vi "MB Serial Call Wait on Query.vi"(9 "Timeout":u32=10000, 10 "Serial Parameters":T1 {"Slave Address" format="%.0x"}, 11 "VISA resource name":refnum<visa-resource-name>) -> ()   [LabVIEW 2011]
panel:
  # "VI Name: MB Serial Call Wait on Query.vi\nPurpose: Dynamically calls MB Serial Wait on Query.vi"
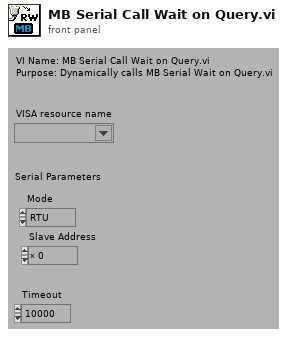
[diagram p1: front panel]
types:
  T1 = cluster{"Mode":enum16{"RTU", "ASCII"}, "Slave Address":u8}
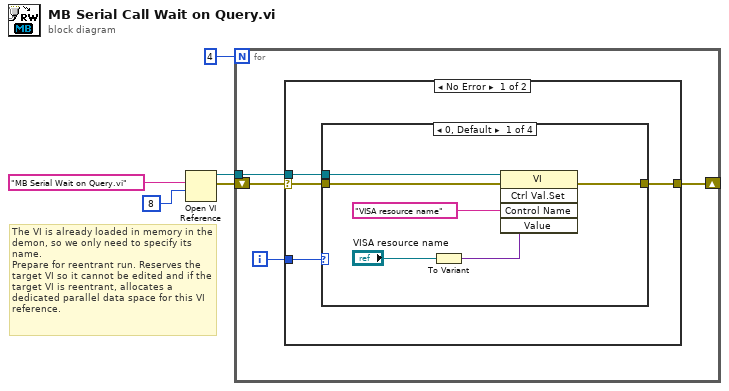
[diagram p0: block diagram]
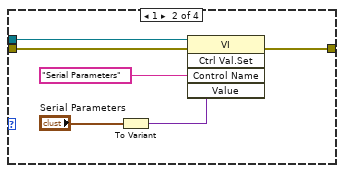
[diagram p2: hidden frame]
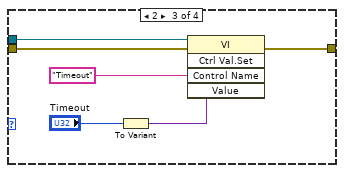
[diagram p3: hidden frame]
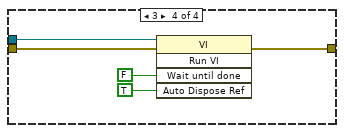
[diagram p4: hidden frame]
diagram:
  # "The VI is already loaded in memory in the demon, so we only need to specify its name.\nPrepare for reentrant run. Reserves the target VI so it cannot be edited and if the target VI is reentrant, allocates a dedicated parallel data space for this VI reference."
  n1 = Open VI Reference(vi path="MB Serial Wait on Query.vi", options=8) -> (vi reference=w5:refnum<vi>, error out=w4:errorcluster)  [unwired: 1 in, 3 out]
  n2 = for {
    N: 4 -> [_]
    tunnel: w5 -> [w9]
    shift-right: [w8] -> _
    shift-left: w4 -> [w7]
    i -> [w6]
    n3 = case shown="No Error" w7 {
      selector: w7 -> [w11 w37]
      tunnel: w9 -> [w13 _]
      tunnel: [w12 w37] -> w8
      tunnel: w6 -> [w10 _]
      frame No Error {
        n4 = case shown="0, Default" w10 {
          tunnel: w13 -> [w19 w25 w31 w36]
          tunnel: w11 -> [w16 w22 w28 w35]
          tunnel: [w15 w21 w27 w34] -> w12
          frame 0, Default {
            n5 = To Variant(anything="VISA resource name") -> (Variant=w17:variant)
            n6 = invoke class="VI" method="Ctrl Val.Set"(reference=w19, error in=w16, "Control Name"="VISA resource name", "Value"=w17) -> (error out=w15:errorcluster)  [unwired: 1 in, 4 out]
          }
          frame 1 {
            n7 = To Variant(anything="Serial Parameters") -> (Variant=w23:variant)
            n8 = invoke class="VI" method="Ctrl Val.Set"(reference=w25, error in=w22, "Control Name"="Serial Parameters", "Value"=w23) -> (error out=w21:errorcluster)  [unwired: 1 in, 4 out]
          }
          frame 2 {
            n9 = To Variant(anything="Timeout") -> (Variant=w29:variant)
            n10 = invoke class="VI" method="Ctrl Val.Set"(reference=w31, error in=w28, "Control Name"="Timeout", "Value"=w29) -> (error out=w27:errorcluster)  [unwired: 1 in, 4 out]
          }
          frame 3 {
            n11 = invoke class="VI" method="Run VI"(reference=w36, error in=w35, "Wait until done"=FALSE, "Auto Dispose Ref"=TRUE) -> (error out=w34:errorcluster)  [unwired: 1 in, 4 out]
          }
        }
      }
      frame Error {
      }
    }
  }
